vi "Analog Read Pin Example.vi"() -> ()   [LabVIEW 2010, in "LabVIEW Interface for Arduino.lvlib"]
doc: "An example that reads a user selectable analog input pin on the Arduino."
uses:
  <vilib>/LabVIEW Interface for Arduino/LabVIEW Interface for Arduino.lvlib
  <vilib>/LabVIEW Interface for Arduino/Type Defs/Analog Pin.ctl
panel:
  in  "Set Function":bool
  in  "Select Function":T1
  in  "Stop":bool
  out "Voltage":dbl(knob) scale=0.0..5.0
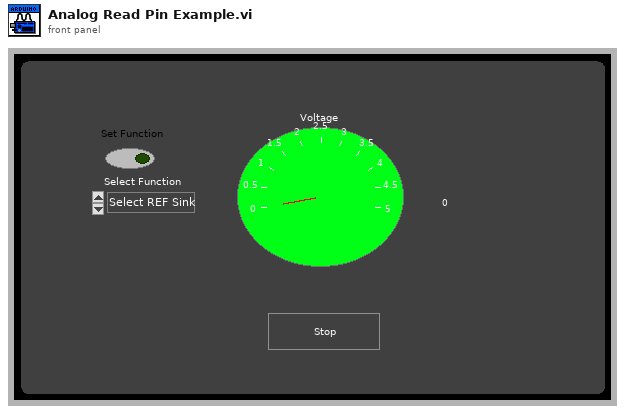
[diagram p1: front panel]
types:
  T1 = typedef "LabVIEW Interface for Arduino.lvlib/Analog Pin.ctl" = enum8{"Select REF Sink", "SelectDUT Sink", "Enable PROG", "Disable PROG", "Enable Register", "Disable Register"}
  T2 = typedef "LabVIEW Interface for Arduino.lvlib/Arduino Resource.ctl" = cluster{"VISA resource":refnum<visa-resource-name>, "Board Type":T3, "Connection Type":enum8{"USB / Serial"}, "Bytes Per Packet (15)":u8}
  T3 = typedef "LabVIEW Interface for Arduino.lvlib/Board Type.ctl" = enum16{"Uno", "Dimuelanove w/Atmega 328", "Mega 2560"}
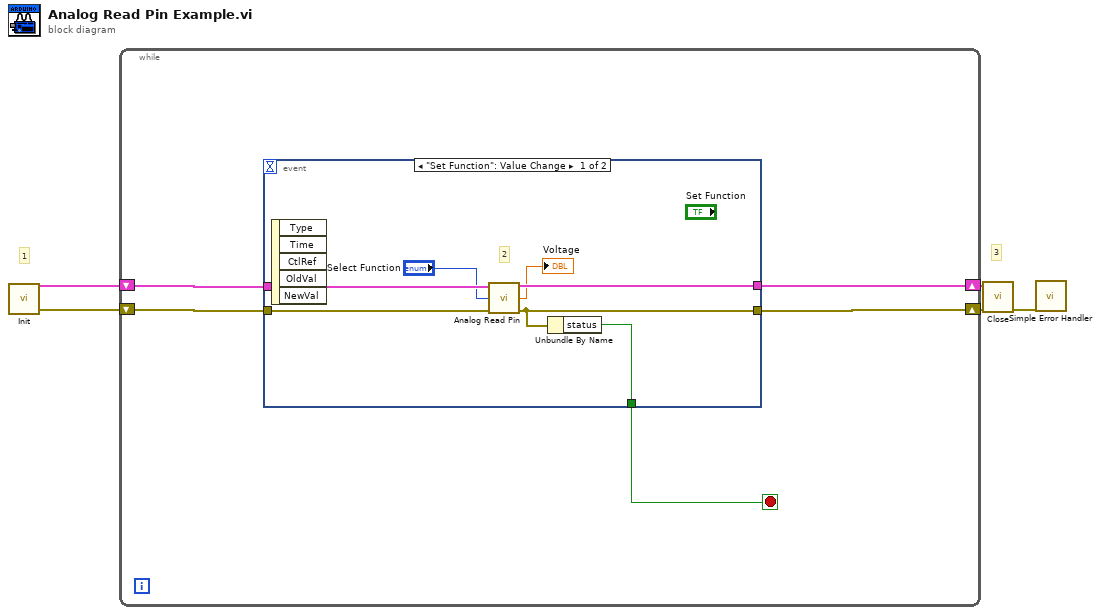
[diagram p0: block diagram]
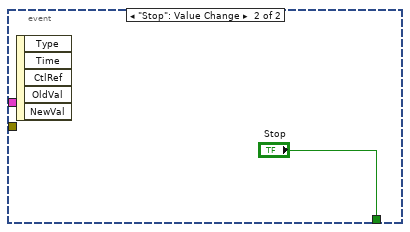
[diagram p2: hidden frame]
diagram:
  # "3"
  # "1"
  n1 = call <vilib>:"Init.vi"() -> ("Arduino Resource"=w5:T2, "error out"=w2:errorcluster)  [unwired: 18 in]
  n2 = while {
    shift-right: [w10] -> w4
    shift-left: w5 -> [w7]
    shift-right: [w9] -> w3
    shift-left: w2 -> [w6]
    stop <- w8 stop-if-true
    n3 = event shown="[0] \"Set Function\": Value Change" {
      selector: _ -> [_ _]
      dyn-events: _ -> [_ _]
      timeout: _ -> [_ _]
      tunnel: [w17 _] -> w10
      tunnel: [w15 _] -> w9
      tunnel: [w11 "Stop"] -> w8
      tunnel: w7 -> [w14 _]
      tunnel: w6 -> [w13 _]
      event "Set Function": Value Change {
        # "2"
        n4 = event-data() -> ()  [unwired: 1 in, 5 out]
        n5 = call <vilib>:"Analog Read Pin.vi"("Arduino Resource"=w14, "Analog Input Pin (0)"="Select Function", "error in"=w13) -> ("Arduino Resource"=w17:T2, "Voltage"=→"Voltage":dbl, "error out"=w15:errorcluster)  [unwired: 10 in]
        n6 = Unbundle By Name(w15) -> ("status"=w11:bool)
      }
      event "Stop": Value Change {
        n7 = event-data() -> ()  [unwired: 1 in, 5 out]
      }
    }
  }
  n8 = call <vilib>:"Close.vi"("Arduino Resource"=w4, "error in"=w3) -> ("error out"=w1:errorcluster)  [unwired: 13 in]
  n9 = call <vilib>:"Simple Error Handler.vi"("error in (no error)"=w1) -> ()  [unwired: 4 in, 5 out]
